vi "TSM SSC DAQmx Write (Analog 1D Wfm) Per-Site Per-Pin.vi"(0 "DAQ TSM in":T1, 1 "Idle Channel Value (0)":dbl, 5 "Per-Site Per-Pin Waveforms in":waveform(dbl)[][](array[waveform]), 11 "error in":errorcluster) -> (4 "DAQ TSM Out":T1, 15 "error out":errorcluster)   [LabVIEW 2020]
doc: "Writes one or more waveforms to a task that contains one or more analog output channels. The waveform data should be in the same order as SSC."
uses:
  Pin Map/TSM DAQmx Multi-Task.ctl
  <vilib>/NI_TestStand_SemiconductorModule/NI_TestStand_Semiconductor_Module.lvlibp/PinMap/PinQueryContext/MultiplePinMultipleSessionQueryContext/MultiplePinMultipleSessionQueryContext.lvclass
  Pin Map/SSC DAQmx.ctl
  523e543d-0678-41ee-875f-de7ba3d8a92e.vi
  <vilib>/DAQmx/write.llb/DAQmx Write (Analog 1D Wfm NChan NSamp).vi
  <vilib>/DAQmx/miscellaneous.llb/DAQmx Fill In Error Info.vi
  <resource>/objmgr/daqmx.rc
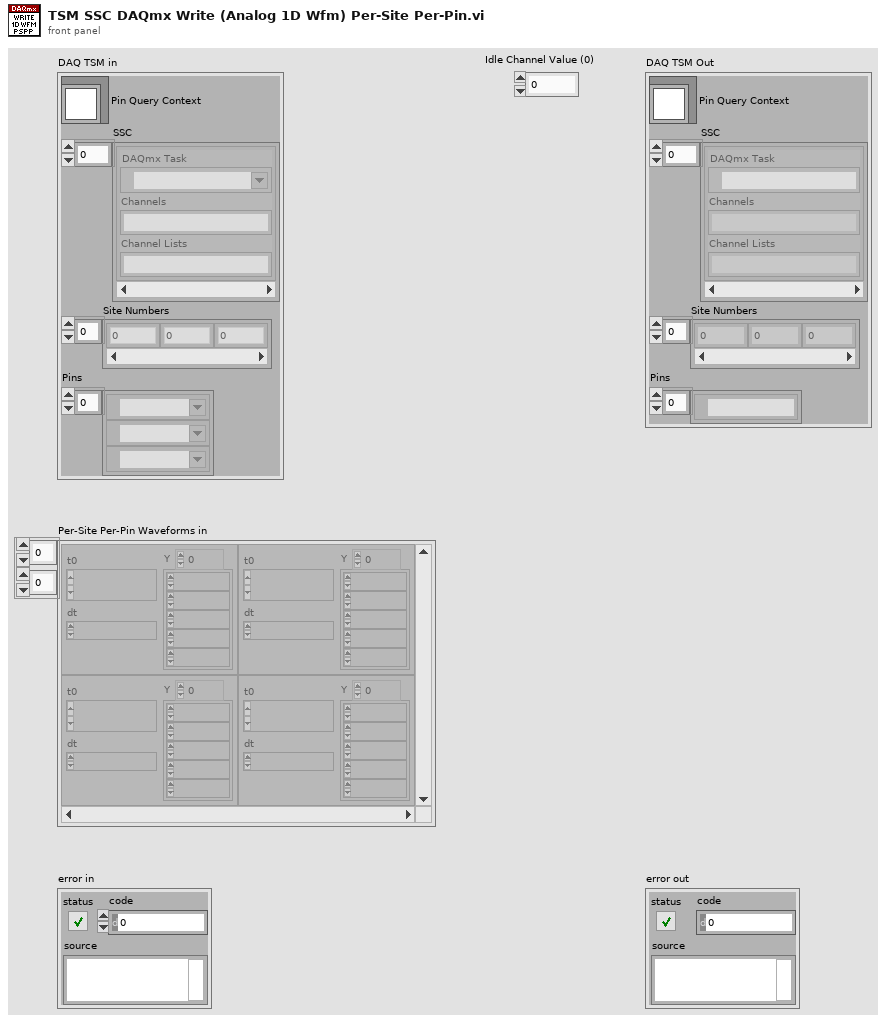
[diagram p1: front panel]
types:
  T1 = typedef "TSM DAQmx Multi-Task.ctl" = cluster{"Pin Query Context":refnum<class "MultiplePinMultipleSessionQueryContext.lvclass">, "SSC":T2[], "Site Numbers":i32[], "Pins":tag[]}
  T2 = typedef "SSC DAQmx.ctl" = cluster{"DAQmx Task ":refnum<k21>, "Channels":string, "Channel Lists":string}
  T3 = typedef "Digital 2D Location.ctl" = cluster{"Row":i32, "Col":i32}
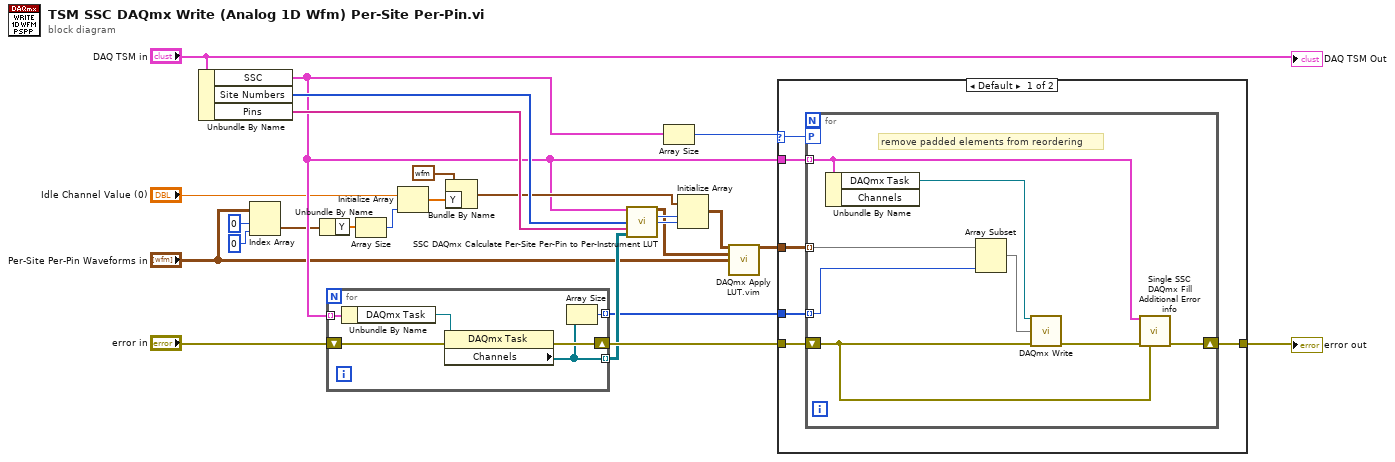
[diagram p0: block diagram]
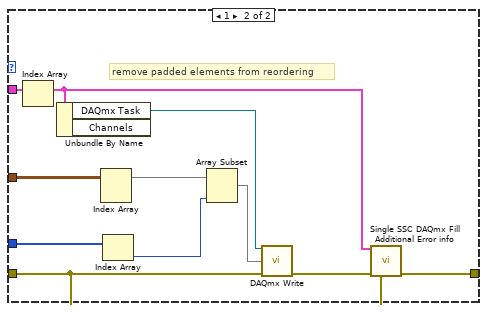
[diagram p2: hidden frame]
diagram:
  n1 = Unbundle By Name("DAQ TSM in") -> ("SSC"=w11:T2[], "Site Numbers"=w22:i32[], "Pins"=w21:tag[])
  n2 = Index Array(array="Per-Site Per-Pin Waveforms in", index (row)=0, index (col)=0 ("disabled index (col)")) -> (element=w6:waveform(dbl))
  n3 = Unbundle By Name(w6) -> ("Y"=w5:dbl[])
  n4 = for {
    shift-right: [w30] -> w12
    shift-left: "error in" -> [w31]
    tunnel: w11 -> [w29] mode=indexing
    tunnel: [w27] -> w10 mode=indexing
    tunnel: [w26] -> w9 mode=indexing
    n5 = Unbundle By Name(w29) -> ("DAQmx Task"=w28:refnum<k21>)
    n6 = property class="DAQmx Task"(reference=w28, error in=w31) -> (error out=w30:errorcluster, "Channels"=w27:refnum<k21>[])  [unwired: 1 out]
    n7 = Array Size(array=w27) -> (size(s)=w26:i32)
  }
  n8 = Array Size(array=w5) -> (size(s)=w4:i32)
  n9 = Initialize Array("Idle Channel Value (0)", w4) -> (w1:dbl[])
  n10 = Bundle By Name ("Build Waveform")(cluster=waveform(dbl) {"t0"=timestamp(0 s since 1904-01-01), "dt"=1.0, "Y"=[0.0]} ("Per-Site Per-Pin Waveforms in"), "Y"=w1) -> (w13:waveform(dbl))
  n11 = call "SSC DAQmx Calculate Per-Site Per-Pin to Per-Instrument LUT.vi"("DAQmx SSC in"=w11, "Sites"=w22, "Pins"=w21, "AO Channels"=w10) -> ("Per-Site Per-Pin to Per-Task LUT"=w18:T3[][], "Task Count"=w20:i32, "Max Channels in a Task"=w19:i32)  [unwired: 9 in]
  n12 = Array Size(array=w11) -> (size(s)=w15:i32)
  n13 = Initialize Array(w13, w20, w19) -> (w17:waveform(dbl)[][])
  n14 = call "DAQmx Apply LUT.vim"("Initialized Array"=w17, "LUT"=w18, "Results to Apply LUT to"="Per-Site Per-Pin Waveforms in") -> ("Array Out"=w16:waveform(dbl)[][])  [unwired: 12 in]
  n15 = case shown="Default" w15 {
    selector: w15 -> [w35 _]
    tunnel: [w37 w56] -> w23
    tunnel: w12 -> [w36 w55]
    tunnel: w11 -> [w34 w54]
    tunnel: w16 -> [w33 w53]
    tunnel: w9 -> [w32 w52]
    frame Default {
      n16 = for {
        tunnel: w34 -> [w42] mode=indexing
        workers-P: w35 -> [_]
        shift-right: [w45] -> w37
        shift-left: w36 -> [w44]
        tunnel: w33 -> [w40] mode=indexing
        tunnel: w32 -> [w38] mode=indexing
        # "remove padded elements from reordering"
        n17 = Unbundle By Name(w42) -> ("DAQmx Task"=w41:refnum<k21>)  [unwired: 1 out]
        n18 = Array Subset(array=w40, length=w38) -> (w39:waveform(dbl)[])  [unwired: 1 in]
        n19 = call-poly <vilib>:"DAQmx Write.vi"("task/channels in"=w41, "data"=w39, "error in"=w44) -> ("error out"=w43:errorcluster)  [unwired: 10 in, 2 out]
        n20 = call "Single SSC DAQmx Fill Additional Error info.vi"("DAQmx SSC in"=w42, "error in"=w43, "previous error in"=w44) -> ("error out"=w45:errorcluster)  [unwired: 12 in]
      }
    }
    frame 1 {
      # "remove padded elements from reordering"
      n21 = Index Array(array=w54) -> (element=w48:T2)  [unwired: 1 in]
      n22 = Unbundle By Name(w48) -> ("DAQmx Task"=w50:refnum<k21>)  [unwired: 1 out]
      n23 = Index Array(array=w53) -> (element=w46:waveform(dbl)[])  [unwired: 2 in]
      n24 = Index Array(array=w52) -> (element=w47:i32)  [unwired: 1 in]
      n25 = Array Subset(array=w46, length=w47) -> (w49:waveform(dbl)[])  [unwired: 1 in]
      n26 = call-poly <vilib>:"DAQmx Write.vi"("task/channels in"=w50, "data"=w49, "error in"=w55) -> ("error out"=w51:errorcluster)  [unwired: 10 in, 2 out]
      n27 = call "Single SSC DAQmx Fill Additional Error info.vi"("DAQmx SSC in"=w48, "error in"=w51, "previous error in"=w55) -> ("error out"=w56:errorcluster)  [unwired: 12 in]
    }
  }
  "error out" <- w23
  "DAQ TSM Out" <- "DAQ TSM in"
